vi "SPCNT Sample.vi"() -> ()   [LabVIEW 2009]
panel:
  out "Frequency [Hz]":dbl caption="Frequency"
  in  "Bin width [ms]":u32 caption="Width"
  in  "?":bool
  # "SPCNT Example"
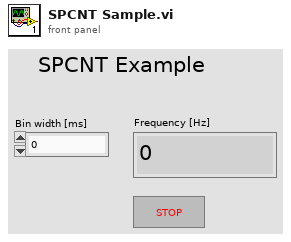
[diagram p1: front panel]
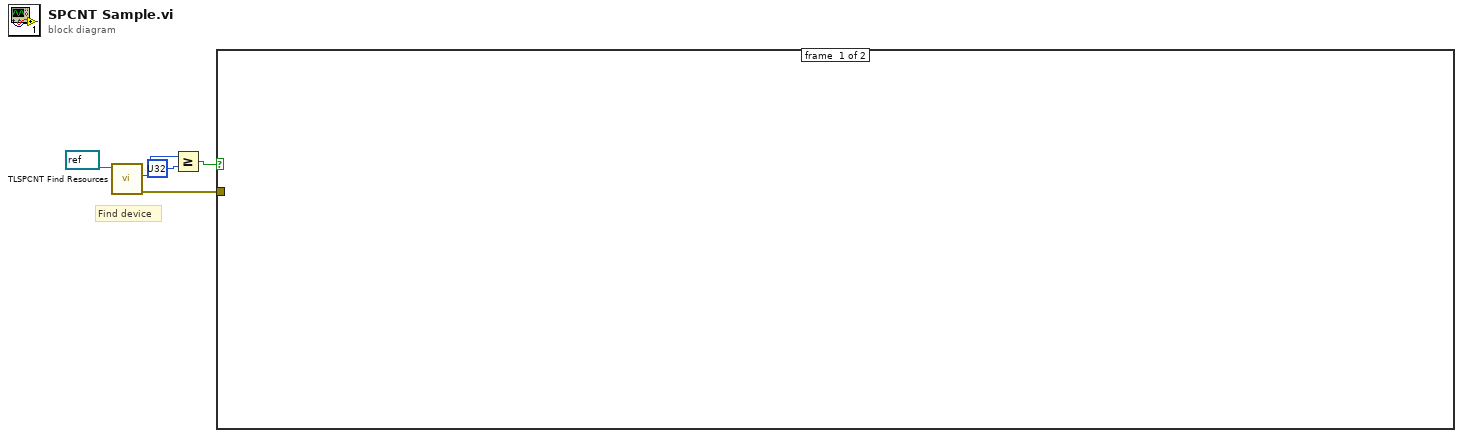
[diagram p0: block diagram]
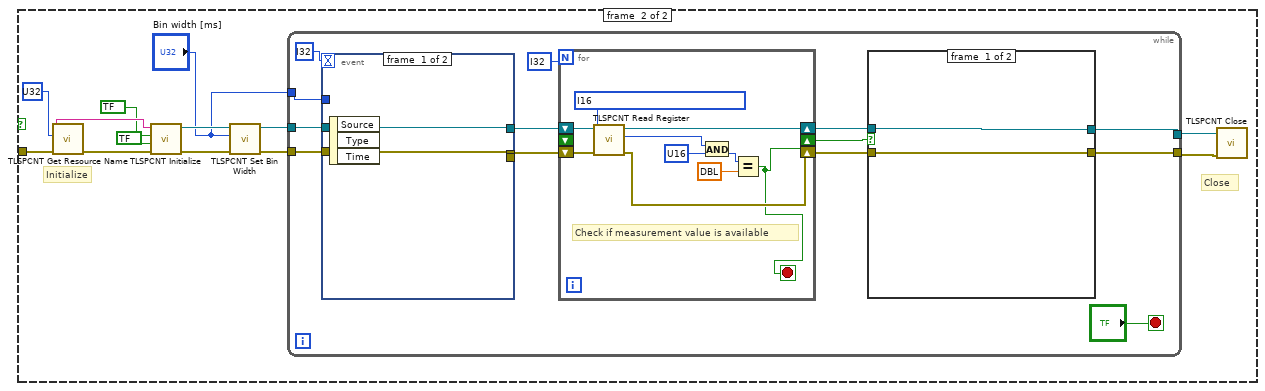
[diagram p2: hidden frame]
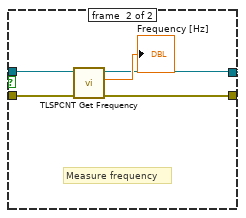
[diagram p3: hidden frame]
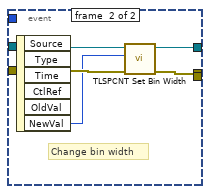
[diagram p4: hidden frame]
diagram:
  # "Find device"
  n1 = call "TLSPCNT Find Resources.vi"("instrument handle"=refnum<visa-resource-name> ?) -> ("error out"=w1:errorcluster, "Resource Count"=w4:u32)  [unwired: 8 in, 1 out]
  n2 = Greater Or Equal?(x=w4, y=u32 ?) -> (x >= y?=w2:bool)
  n3 = case shown="True" w2 {
    tunnel: w1 -> [_ w18]
    frame #0 {
    }
    frame #1 {
      # "Close"
      # "Initialize"
      n4 = call "TLSPCNT Get Resource Name.vi"("error in (no error)"=w18, "Index (0)"=u32 ?) -> ("error out"=w13:errorcluster, "Resource Name"=w16:string)  [unwired: 7 in, 1 out]
      n5 = call "TLSPCNT Initialize.vi"("error in (no error)"=w13, "Reset Device (Yes)"=bool ?, "ID Query (Yes)"=bool ?, "resource name"=w16) -> ("error out"=w9:errorcluster, "instrument handle out"=w10:refnum<visa-resource-name>)  [unwired: 6 in]
      n6 = call "TLSPCNT Set Bin Width.vi"("error in (no error)"=w9, "Width"="Bin width [ms]", "instrument handle"=w10) -> ("error out"=w7:errorcluster, "instrument handle out"=w8:refnum<visa-resource-name>)  [unwired: 7 in]
      n7 = while {
        tunnel: [w28] -> w12
        tunnel: "Bin width [ms]" -> [w23]
        tunnel: [w24] -> w11
        tunnel: w8 -> [w21]
        tunnel: w7 -> [w20]
        stop <- "?" stop-if-true
        n8 = event shown="[1] \"Bin width [ms]\": Value Change" {
          selector: _ -> [_ _]
          dyn-events: _ -> [_ _]
          timeout: i32 ? -> [_ _]
          tunnel: w21 -> [w50 w55]
          tunnel: w20 -> [w49 w54]
          tunnel: [w50 w52] -> w27
          tunnel: [_ w51] -> w26
          tunnel: [w49 _] -> _
          tunnel: w23 -> [_ _]
          event #0 {
            n9 = event-data() -> ()  [unwired: 1 in, 3 out]
          }
          event #1 {
            # "Change bin width"
            n10 = event-data() -> ("NewVal"=w53:u32)  [unwired: 1 in, 5 out]
            n11 = call "TLSPCNT Set Bin Width.vi"("error in (no error)"=w54, "Width"=w53, "instrument handle"=w55) -> ("error out"=w51:errorcluster, "instrument handle out"=w52:refnum<visa-resource-name>)  [unwired: 7 in]
          }
        }
        n12 = for {
          N: i32 ? -> [_]
          shift-right: [w44] -> w30
          shift-left: w27 -> [w48]
          shift-right: [w46] -> w29
          shift-left: w26 -> [w47]
          shift-right: [w39] -> w19
          shift-left: _ -> [_]
          stop <- w39 stop-if-true
          w45 = i16 ? items=["Service Request Enable", "Standard Event Enable", "Operation Event Register", "Operation Condition Register", "Operation Enable Register", "Operation Positive Transition Filter", "Operation Negative Transition Filter", "Questionable Event Register", "Questionable Condition Register", "Questionable Enable Register", "Questionable Positive Transition Filter", "Questionable Negative Transition Filter"] ("Register ID (Service Request Enable)")
          # "Check if measurement value is available"
          n13 = call "TLSPCNT Read Register.vi"("error in (no error)"=w47, "Register ID (Service Request Enable)"=w45, "instrument handle"=w48) -> ("error out"=w46:errorcluster, "Value"=w42:u16, "instrument handle out"=w44:refnum<visa-resource-name>)  [unwired: 6 in]
          n14 = And(x=w42, y=u16 ?) -> (x .and. y?=w40:u16)
          n15 = Equal?(x=w40, y=dbl ?) -> (x = y?=w39:bool)
        }
        n16 = case shown="True" w19 {
          tunnel: w30 -> [w33 w35]
          tunnel: w29 -> [w32 w34]
          tunnel: [w33 w37] -> w28
          tunnel: [w32 w36] -> w24
          frame #0 {
          }
          frame #1 {
            # "Measure frequency"
            n17 = call "TLSPCNT Get Frequency.vi"("error in (no error)"=w34, "instrument handle"=w35) -> ("error out"=w36:errorcluster, "Frequency"=→"Frequency [Hz]":dbl, "instrument handle out"=w37:refnum<visa-resource-name>)  [unwired: 4 in, 3 out]
          }
        }
      }
      n18 = call "TLSPCNT Close.vi"("error in (no error)"=w11, "instrument handle"=w12) -> ()  [unwired: 9 in, 1 out]
    }
  }
